vi "Create.vi"(8 "error in":errorcluster, 10 "Config Files Directory":path) -> (0 "error out":errorcluster, 3 "Config Manager out":refnum<class "Config Manager Class.lvclass">)   [LabVIEW 2011, in "Config Manager Class.lvclass"]
uses:
  Config Manager Class.lvclass
  Config Manager Class.lvclass/Config Manager Class.ctl
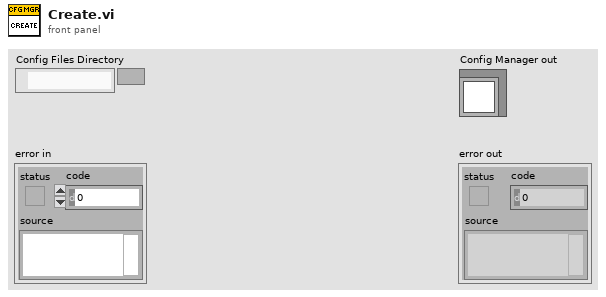
[diagram p1: front panel]
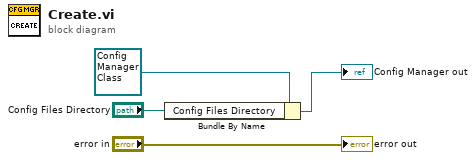
[diagram p0: block diagram]
diagram:
  n1 = Bundle By Name(cluster=refnum<class "Config Manager Class.lvclass"> refnum ("Config Manager Class in"), "Config Files Directory"="Config Files Directory") -> (→"Config Manager out":refnum<class "Config Manager Class.lvclass">)
  "error out" <- "error in"
